vi "Check For Error.vi"(8 "error in (no error)":errorcluster, 11 "configuration session error":T1) -> (0 "error out":errorcluster, 3 "is error?":bool)   [LabVIEW 2019, in "DSF Core.lvlib" / "Configuration Session.lvclass"]
uses:
  Configuration Session.lvclass
  Errors.ctl
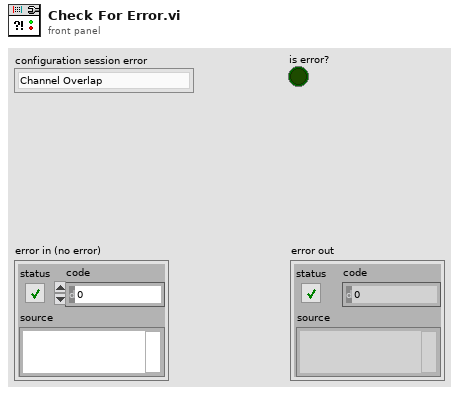
[diagram p1: front panel]
types:
  T1 = typedef "DSF Core.lvlib/Configuration Session.lvclass/Errors.ctl" = enum16{"Channel Overlap", "Invalid Engine Offset", "Invalid JSON"}
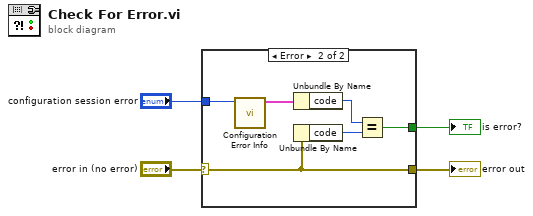
[diagram p0: block diagram]
diagram:
  n1 = case shown="Error" "error in (no error)" {
    selector: "error in (no error)" -> [w5 w9]
    tunnel: "configuration session error" -> [_ w11]
    tunnel: [w5 w9] -> w2
    tunnel: [_ w6] -> w1
    frame No Error {
    }
    frame Error {
      n2 = call "Configuration Error Info.vi"("configuration error"=w11) -> ("error info"=w10:cluster{"code":i32, "description":string})  [unwired: 10 in]
      n3 = Unbundle By Name(w10) -> ("code"=w7:i32)
      n4 = Unbundle By Name(w9) -> ("code"=w8:i32)
      n5 = Equal?(x=w7, y=w8) -> (x = y?=w6:bool)
    }
  }
  "error out" <- w2
  "is error?" <- w1
